vi "Signal mixer.vi"(0 "source A":dbl, 7 "combo mode":bool, 11 "source B":dbl) -> (8 "output":dbl)   [LabVIEW 2019]
doc: "This subvi adds or multiplies two signals on a point by point basis.\n\nIf one of the inputs is zero, it is replaced by 1 in the multiplication.\n\nPaul K Dixon\nP3600\nCSUSB Physics"
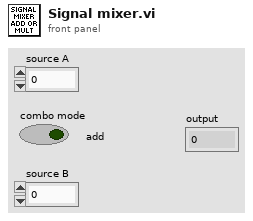
[diagram p1: front panel]
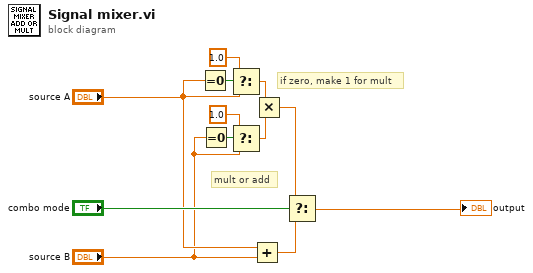
[diagram p0: block diagram]
diagram:
  # "mult or add"
  # "if zero, make 1 for mult"
  n1 = Equal To 0?(x="source A") -> (x = 0?=w9:bool)
  n2 = Equal To 0?(x="source B") -> (x = 0?=w5:bool)
  n3 = Select(t=1.0, s=w9, f="source A") -> (s? t:f=w8:dbl)
  n4 = Select(t=1.0, s=w5, f="source B") -> (s? t:f=w4:dbl)
  n5 = Add(x="source A", y="source B") -> (x+y=w11:dbl)
  n6 = Multiply(x=w8, y=w4) -> (x*y=w12:dbl)
  n7 = Select(t=w12, s="combo mode", f=w11) -> (s? t:f=→"output":dbl)
